vi "MaxSearch.vi"(0 "DataArray":dbl[][](array[numeric])=[[30.5, 10.0, 0.0, 0.0, 100.0], [30.5, 11.0, 0.0, 0.0, 300.0], [30.5, 12.0, 0.0, 0.0, 100.0], [31.5, 10.0, 0.0, 0.0, 110.0], [31.5, 11.0, 0.0, 0.0, 310.0], [31.5, 12.0, 0.0, 0.0, 110.0], [32.5, 10.0, 0.0, 0.0, 100.0], [32.5, 11.0, 0.0, 0.0, 300.0], [32.5, 12.0, 0.0, 0.0, 100.0], [nan, nan, 0.0, 0.0, nan], [14.5, 10.0, 0.0, 0.0, 100.0], [14.5, 11.0, 0.0, 0.0, 300.0], [14.5, 12.0, 0.0, 0.0, 100.0], [15.5, 10.0, 0.0, 0.0, 110.0], [15.5, 11.0, 0.0, 0.0, 310.0], [15.5, 12.0, 0.0, 0.0, 110.0], [16.5, 10.0, 0.0, 0.0, 100.0], [16.5, 11.0, 0.0, 0.0, 300.0], [16.5, 12.0, 0.0, 0.0, 100.0]]) -> (1 "MaxData":dbl[][](array[numeric]), 2 "Center":cluster{dbl, dbl, dbl})   [LabVIEW 2014]
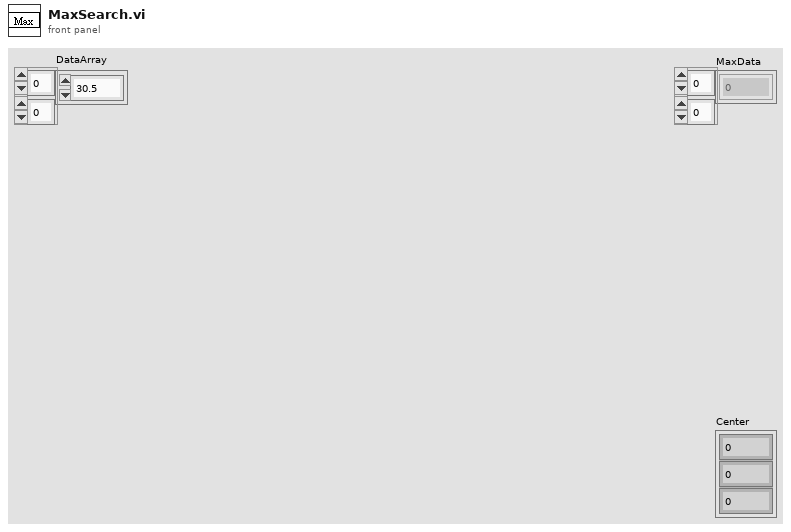
[diagram p1: front panel]
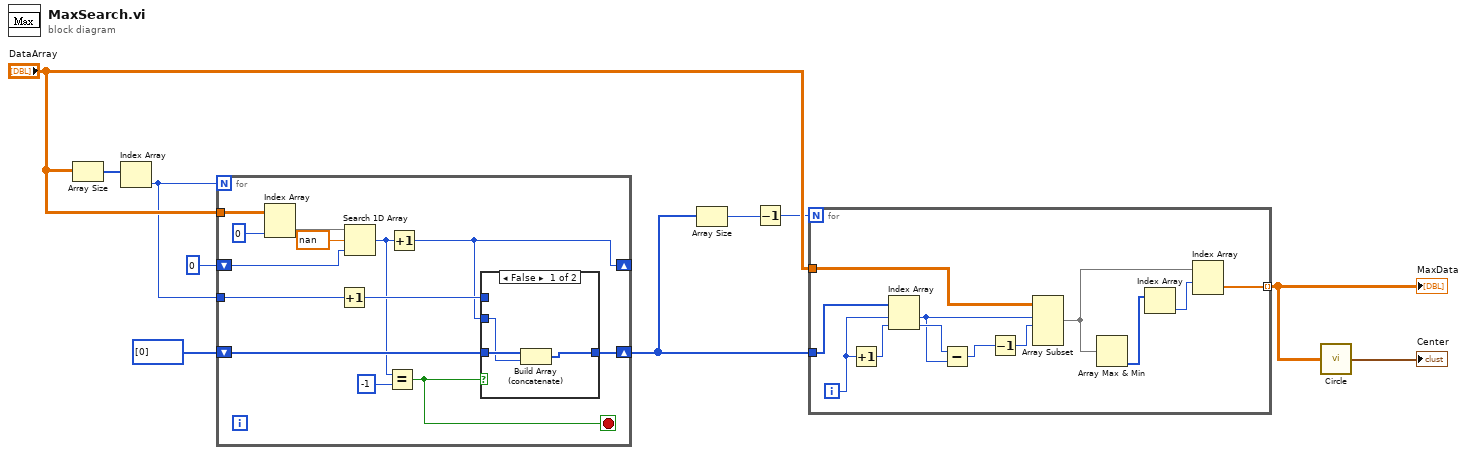
[diagram p0: block diagram]
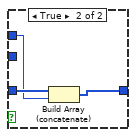
[diagram p2: hidden frame]
diagram:
  n1 = Array Size(array="DataArray") -> (size(s)=w10:i32[])
  n2 = Index Array(array=w10) -> (element=w3:i32)  [unwired: 1 in]
  n3 = for {
    N: w3 -> [_]
    shift-right: [w17] -> w6
    shift-left: i32[] [0] -> [w18]
    shift-right: [w12] -> _
    shift-left: 0 -> [w16]
    tunnel: "DataArray" -> [w20]
    tunnel: w3 -> [w15]
    stop <- w11 stop-if-true
    n4 = Index Array(array=w20, index (col)=0 ("disabled index (col)")) -> (element=w23:dbl[])  [unwired: 1 in]
    n5 = Increment(x=w15) -> (x+1=w14:i32)
    n6 = Search 1D Array(1D array=w23, element=nan, start index (0)=w16) -> (index of element=w13:i32)
    n7 = Equal?(x=w13, y=-1) -> (x = y?=w11:bool)
    n8 = Increment(x=w13) -> (x+1=w12:i32)
    n9 = case shown="False" w11 {
      tunnel: w18 -> [w26 w28]
      tunnel: [w25 w29] -> w17
      tunnel: w12 -> [w24 _]
      tunnel: w14 -> [_ w27]
      frame False {
        n10 = Build Array (concatenate)(w26, w24) -> (w25:i32[])
      }
      frame True {
        n11 = Build Array (concatenate)(w28, w27) -> (w29:i32[])
      }
    }
  }
  n12 = Array Size(array=w6) -> (size(s)=w7:i32)
  n13 = Decrement(x=w7) -> (x-1=w5:i32)
  n14 = for {
    N: w5 -> [_]
    tunnel: "DataArray" -> [w41]
    tunnel: w6 -> [w40]
    tunnel: [w36] -> w2 mode=indexing
    i -> [w38]
    n15 = Increment(x=w38) -> (x+1=w39:i32)
    n16 = Index Array(array=w40, index #1=w38, index #2=w39) -> (element #1=w33:i32, element #2=w34:i32)
    n17 = Subtract(x=w34, y=w33) -> (x-y=w32:i32)
    n18 = Decrement(x=w32) -> (x-1=w31:i32)
    n19 = Array Subset(array=w41, index (row)=w33, length (row)=w31) -> (w35:dbl[][])  [unwired: 2 in]
    n20 = Array Max & Min(array=w35) -> (min index (indices)=w30:i32[])  [unwired: 3 out]
    n21 = Index Array(array=w30) -> (element=w37:i32)  [unwired: 1 in]
    n22 = Index Array(array=w35, index (row)=w37) -> (element=w36:dbl[])  [unwired: 1 in]
  }
  "MaxData" <- w2
  n23 = call "Circle.vi"("MaxArray"=w2) -> ("Center"=→"Center":cluster{dbl, dbl, dbl})
